vi "pressureSensor_run.vi"(8 "error in (no error)":errorcluster, 9 "outer Loop counter":i32, 11 "Initial Settings":T1={"Water density"=1000.0, "SB_parameters"={"x0"=0.0, "U_full"=0.695, "U_empty"=3.67}}) -> (0 "error out":errorcluster)   [LabVIEW 2013]
uses:
  My Computer/Controls/Sensors State.ctl
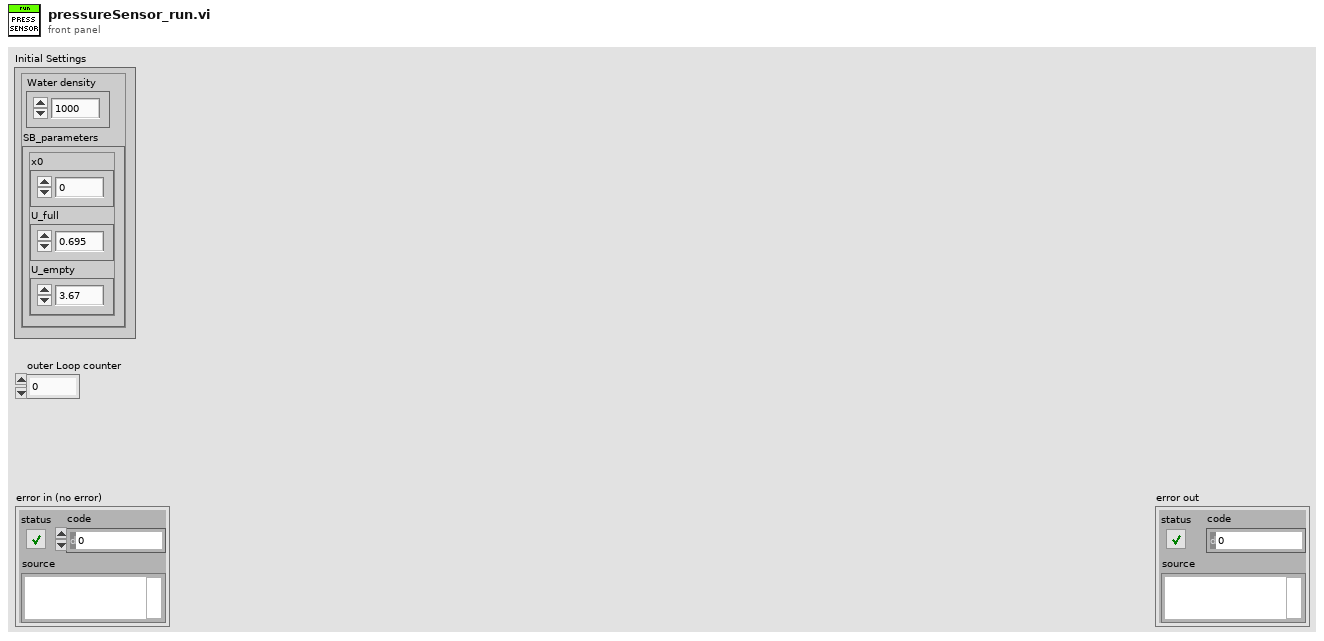
[diagram p1: front panel]
types:
  T1 = cluster{"Water density":dbl, "SB_parameters":cluster{"x0":dbl, "U_full":dbl, "U_empty":dbl}}
  T2 = typedef "Sensors State.ctl" = cluster{"Leakage-Sensor_enabled":bool, "IMU_enabled":bool, "Swimbladder Fill-State-Sensor_enabled":bool, "Flow-Sensor_enabled":bool, "Depth-Sensor_enabled":bool, "Current-Sensor_enabled":bool, "Calibrate Depth":bool, "SB_Piston_Stuck_Detect_enabled":bool, "Check_too_Deep_enabled":bool}
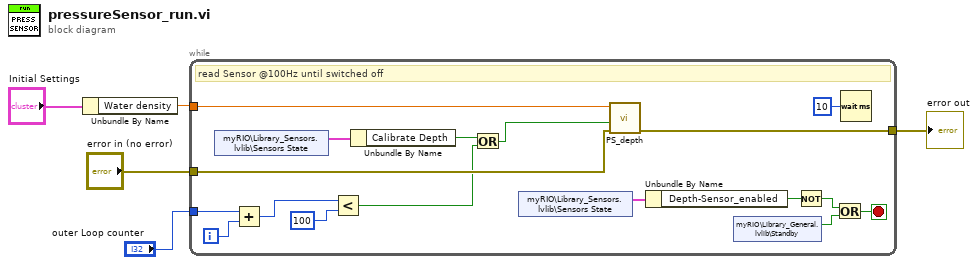
[diagram p0: block diagram]
diagram:
  n1 = Unbundle By Name("Initial Settings") -> ("Water density"=w2:dbl)
  n2 = while {
    tunnel: w2 -> [w18]
    tunnel: "error in (no error)" -> [w17]
    tunnel: [w16] -> w5
    tunnel: "outer Loop counter" -> [w8]
    i -> [w9]
    stop <- w19 stop-if-true
    # "read Sensor @100Hz until switched off"
    n3 = shared-variable "myRIO\\Library_Sensors.lvlib\\Sensors State"() -> (w11:T2)  [unwired: 1 in, 1 out]
    n4 = Add(x=w8, y=w9) -> (x+y=w7:i32)
    n5 = Less?(x=w7, y=100) -> (x < y?=w15:bool)
    n6 = Unbundle By Name(w11) -> ("Calibrate Depth"=w10:bool)
    n7 = Or(x=w10, y=w15) -> (x .or. y?=w14:bool)
    n8 = shared-variable "myRIO\\Library_Sensors.lvlib\\Sensors State"() -> (w13:T2)  [unwired: 1 in, 1 out]
    n9 = call "PS_depth.vi"("error in (no error)"=w17, "Calibrate"=w14, "Water density [kg/m^3]"=w18) -> ("error out"=w16:errorcluster)  [unwired: 1 in, 3 out]
    n10 = Unbundle By Name(w13) -> ("Depth-Sensor_enabled"=w12:bool)
    n11 = shared-variable "myRIO\\Library_General.lvlib\\Standby"() -> (w21:bool)  [unwired: 1 in, 1 out]
    n12 = Not(x=w12) -> (.not. x?=w20:bool)
    n13 = Or(x=w20, y=w21) -> (x .or. y?=w19:bool)
    n14 = Wait (ms)(milliseconds to wait=u32 10) -> ()  [unwired: 1 out]
  }
  "error out" <- w5
